vi "Init.vi"(8 "error in (no error)":errorcluster) -> (0 "error out":errorcluster, 3 "AsyncClassTemplate out":refnum<class "AsyncClassTemplate.lvclass">)   [LabVIEW 2020, in "Vecto.lvlib" / "AsyncClassTemplate.lvclass"]
uses:
  AsyncClassTemplate.lvclass
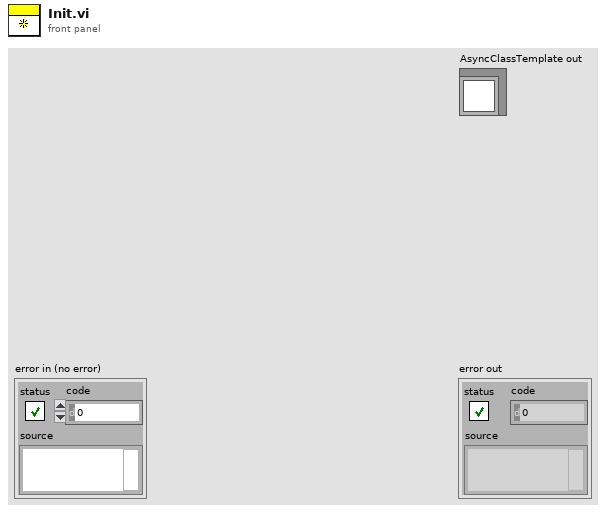
[diagram p1: front panel]
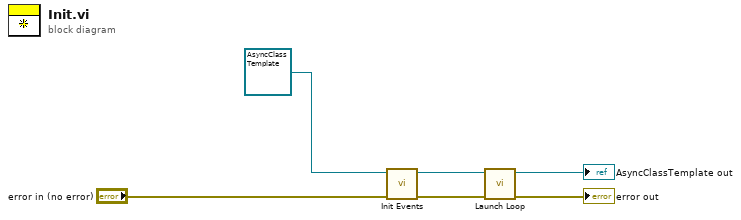
[diagram p0: block diagram]
diagram:
  n1 = call "Init Events.vi"("error in (no error)"="error in (no error)", "AsyncClassTemplate in"=refnum<class "AsyncClassTemplate.lvclass"> refnum) -> ("error out"=w5:errorcluster, "AsyncClassTemplate out"=w2:refnum<class "AsyncClassTemplate.lvclass">)  [unwired: 8 in]
  n2 = call "Launch Loop.vi"("error in (no error)"=w5, "AsyncClassTemplate in"=w2) -> ("error out"=→"error out":errorcluster, "AsyncClassTemplate out"=→"AsyncClassTemplate out":refnum<class "AsyncClassTemplate.lvclass">)  [unwired: 8 in]
